vi "DataFinder_DisplaySignals.vi"(8 "error in":errorcluster {"code" min=0 max=0}, 10 "result references":refnum<k20>[](array[refnum])) -> ()   [LabVIEW 2023]
doc: "Displays resulting signals as waveforms."
uses:
  <vilib>/Utility/error.llb/DialogType.ctl
  <vilib>/DataFinder/Results to Waveforms (ddt).vi
  <vilib>/DataFinder/NI_DataFinder.lvlib
panel:
  out "Resulting Signals":dynamicdata(graph)
  out "error text":string=" INSTRUCTIONS:\r\rNormal Use:  When using subVIs that incorporate the error in/error out (or error I/O) structure, place this handler where you want to inform the user of an error, typically at the end of the I/O data path, as the last action of the program.  If the error in error? is ERROR, the handler creates a message describing the error and its source.  If the type of dialog = 1 (default), the message is displayed to the user, who can only acknowedge it.  If the type = 2, the user can acknowledge the message or abort execution; aborting a program with active I/O is not recommended.  If the type = 0, no message is displayed; this is used to process the error programmatically, and the error out cluster elements are wired to individual terminals for that reason.  \r\rOther Use:\n\r\nlocal testing.  To test the error code of a subVI or function that does not have the error I/O structure, you can wire its error code and a source string to the local error code and error source inputs.  If error in error? indicates no error and error code is not equal to 0, the local code and source are substituted for the error in values, and error? is set TRUE (ERROR)."
  in  "Close":bool
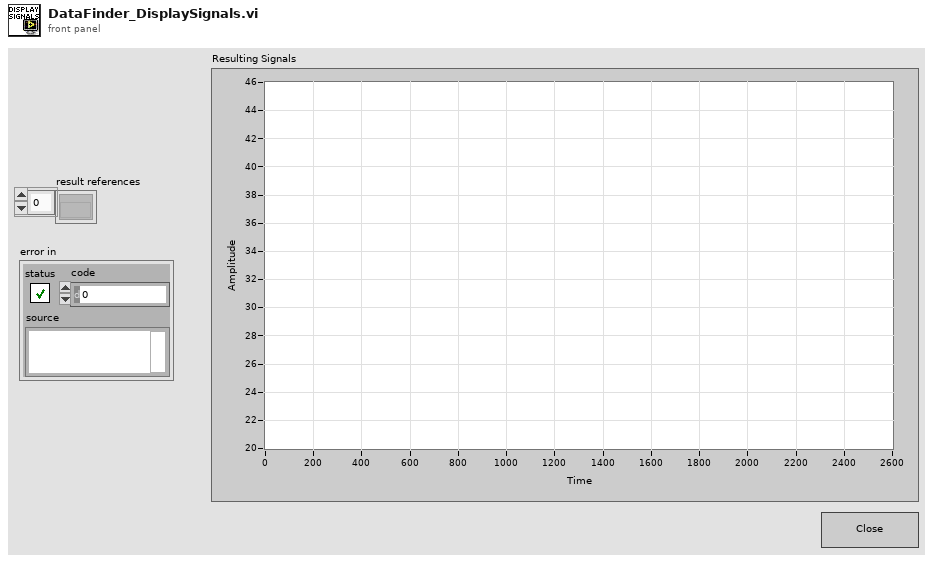
[diagram p1: front panel]
types:
  T1 = typedef "DialogType.ctl" = u16
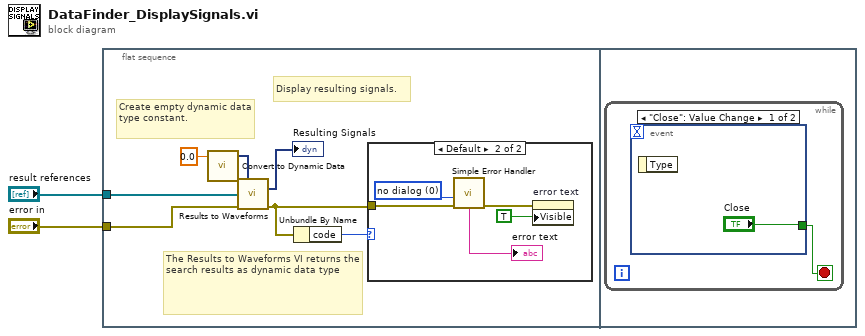
[diagram p0: block diagram]
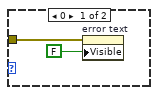
[diagram p2: hidden frame]
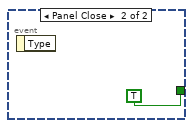
[diagram p3: hidden frame]
diagram:
  n1 = flat-sequence {
    tunnel: "result references" -> [w4]
    tunnel: "error in" -> [w3]
    frame #0 {
      # "The Results to Waveforms VI returns the search results as dynamic data type"
      # "Display resulting signals."
      # "Create empty dynamic data type constant."
      n2 = call "Convert to Dynamic Data"("Double"=0.0) -> ("Dynamic Data Type"=w9:dynamicdata)  [unwired: 3 out]
      n3 = call-poly <vilib>:"Results to Waveforms.vi"("data type"=w9, "result references"=w4, "error in (no error)"=w3) -> ("signals out"=→"Resulting Signals":dynamicdata, "error out"=w7:errorcluster)  [unwired: 10 in, 1 out]
      n4 = Unbundle By Name(w7) -> ("code"=w6:i32)
      n5 = case shown="Default" w6 {
        tunnel: w7 -> [w10 w12]
        frame 0 {
          n6 = property on="error text" class="Str"(error in=w10, "Visible"=FALSE) -> ()  [unwired: 1 in, 2 out]
        }
        frame Default {
          w16 = T1 0 items=["no dialog", "OK message", "continue or stop message", "OK message + warnings", "continue/stop + warnings"] ("type of dialog (OK msg:1)")
          n7 = call <vilib>:"Simple Error Handler.vi"("type of dialog (OK msg:1)"=w16, "error in (no error)"=w12) -> ("error out"=w13:errorcluster, "message"=→"error text":string)  [unwired: 2 in, 4 out]
          n8 = property on="error text" class="Str"(error in=w13, "Visible"=TRUE) -> ()  [unwired: 1 in, 2 out]
        }
      }
    }
    frame #1 {
      n9 = while {
        stop <- w17 stop-if-true
        n10 = event shown="[0] \"Close\": Value Change" {
          selector: _ -> [_ _]
          dyn-events: _ -> [_ _]
          timeout: _ -> [_ _]
          tunnel: ["Close" TRUE ("Cancel")] -> w17
          event "Close": Value Change {
            n11 = event-data() -> ()  [unwired: 1 in, 1 out]
          }
          event Panel Close {
            n12 = event-data() -> ()  [unwired: 1 in, 1 out]
          }
        }
      }
    }
  }
